vi "Decimation.vi"(10 "d":i32=9, 11 "signal in":waveform(dbl)={"t0"=timestamp(0 s since 1904-01-01), "dt"=9.765625e-08, "Y"=array[2000000 elements]}) -> (3 "output waveform":waveform(dbl)={"t0"=timestamp(0 s since 1904-01-01), "dt"=5e-05, "Y"=array[3907 elements]})   [LabVIEW 2019]
uses:
  MeasSNRResults.ctl
  <vilib>/imath/engines/lvmath2/RunTimeEngine/NodeEndStatement/NIMS_NodeEndStatement_Output.vi
  <instcachedir>/0/NIMS_NodeEndStatement_Output_53EC0D466D134D7ABD903AC30B43404B.lvgen/NIMS_NodeEndStatement_Output_53EC0D466D134D7ABD903AC30B43404B_001.vi
  <vilib>/imath/engines/lvmath2/RunTimeEngine/ErrorHandling/NIMS_Finalize Error.vi
  <vilib>/measure/macond.llb/FIR Filter for 1 Chan.vi
  <vilib>/measure/NI_MAPro.lvlib
panel:
  out "MACS/s Total":dbl
  out "MACS/s 2":dbl=418880000.0
  out "MACS/s":dbl=1423360000.0
  out "MeasSNRResults":T1={"VSignalRMS"=3.2614740031076654e-08, "VNoiseRMS"=0.06936052301211641, "SNR(dB)"=-126.55396876238336, "NumBits"=-21.314612751226473, "SNRFS(dB)"=20.167452857912984, "NumBitsFS"=3.05771642158023} {"SNRFS(dB)" format="%_3p"; "NumBitsFS" format="%.1f"; "NumBits" format="%.1f"; "SNR(dB)" format="%_3p"; "VNoiseRMS" format="%#_3p"; "VSignalRMS" format="%#_3p"}
  out "Fs":dbl=10240000.0
  out "FIR filter specifications 2":T2={"Topology"=enum."FIR by Specification", "Type"=enum."Lowpass", "#Taps"=0, "Lower PB"=9000.0, "Upper PB"=0.0, "Lower SB"=10000.0, "Upper SB"=0.0} {"Lower SB" format="%0.2p"; "Upper SB" format="%0.2p"; "Lower PB" format="%0.2p"; "Upper PB" format="%0.2p"}
  out "filter information 2":T3={"magnitude H(w)"={"f0"=0.0, "df"=312.5, "Mag H(w)"=array[513 elements]}, "phase H(w)"={"f0"=0.0, "df"=312.5, "Phase H(w)"=array[513 elements]}, "order"=1309} {"phase H(w)"."df" format="%.2p"; "phase H(w)"."f0" format="%.2p"; "phase H(w)"."Phase H(w)" format="%.2p"; "magnitude H(w)"."df" format="%.2p"; "magnitude H(w)"."f0" format="%.2p"; "magnitude H(w)"."Mag H(w)" format="%.2p"}
  in  "optional FIR filter specifications 2":T4={"PB Gain"=0.087, "SB Gain"=-112.0, "Scale"=TRUE, "Window"=enum."None"} {"SB Gain" format="%.2p"; "PB Gain" format="%.2p"}
  out "filter information":T3={"magnitude H(w)"={"f0"=0.0, "df"=10000.0, "Mag H(w)"=array[513 elements]}, "phase H(w)"={"f0"=0.0, "df"=10000.0, "Phase H(w)"=array[513 elements]}, "order"=139} {"phase H(w)"."df" format="%.2p"; "phase H(w)"."f0" format="%.2p"; "phase H(w)"."Phase H(w)" format="%.2p"; "magnitude H(w)"."df" format="%.2p"; "magnitude H(w)"."f0" format="%.2p"; "magnitude H(w)"."Mag H(w)" format="%.2p"}
  in  "optional FIR filter specifications":T4={"PB Gain"=0.086, "SB Gain"=-112.0, "Scale"=TRUE, "Window"=enum."None"} {"SB Gain" format="%.2p"; "PB Gain" format="%.2p"}
  out "FIR filter specifications":T2={"Topology"=enum."FIR by Specification", "Type"=enum."Lowpass", "#Taps"=0, "Lower PB"=10000.0, "Upper PB"=0.0, "Lower SB"=310000.0, "Upper SB"=0.0} {"Lower SB" format="%0.2p"; "Upper SB" format="%0.2p"; "Lower PB" format="%0.2p"; "Upper PB" format="%0.2p"}
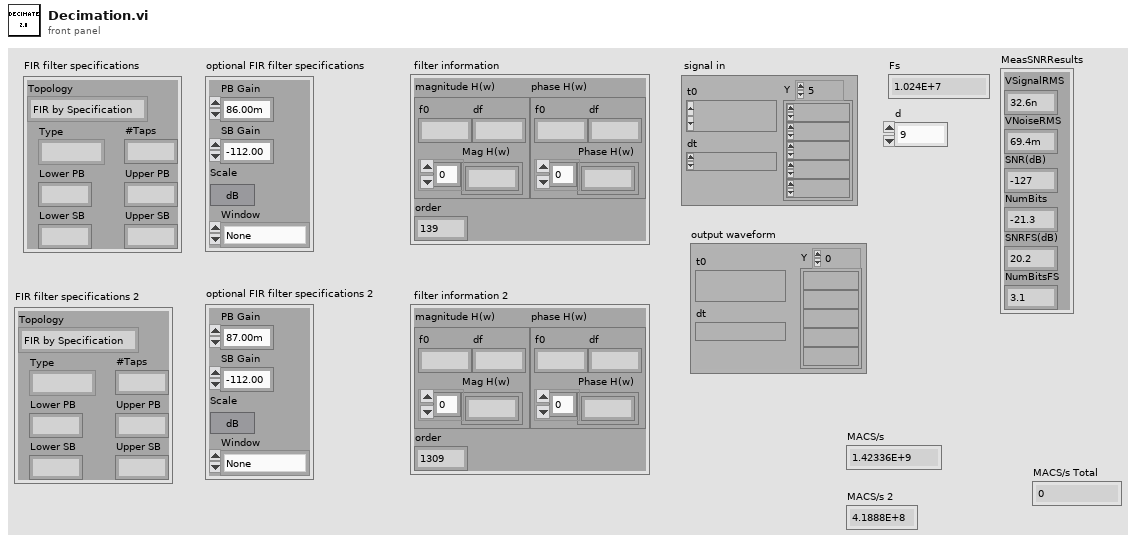
[diagram p1: front panel]
types:
  T1 = typedef "MeasSNRResults.ctl" = cluster{"VSignalRMS":dbl, "VNoiseRMS":dbl, "SNR(dB)":dbl, "NumBits":dbl, "SNRFS(dB)":dbl, "NumBitsFS":dbl}
  T2 = cluster{"Topology":enum16{"Off", "FIR by Specification", "Equi-ripple FIR", "Windowed FIR"}, "Type":enum16{"Lowpass", "Highpass", "Bandpass", "Bandstop"}, "#Taps":i32, "Lower PB":dbl, "Upper PB":dbl, "Lower SB":dbl, "Upper SB":dbl}
  T3 = cluster{"magnitude H(w)":cluster{"f0":dbl, "df":dbl, "Mag H(w)":dbl[]}, "phase H(w)":cluster{"f0":dbl, "df":dbl, "Phase H(w)":dbl[]}, "order":i32}
  T4 = cluster{"PB Gain":dbl, "SB Gain":dbl, "Scale":bool, "Window":enum16{"None", "Hanning", "Hamming", "Triangular", "Blackman", "Exact Blackman", "Blackman-Harris", "Kaiser-Bessel", "Flat Top"}}
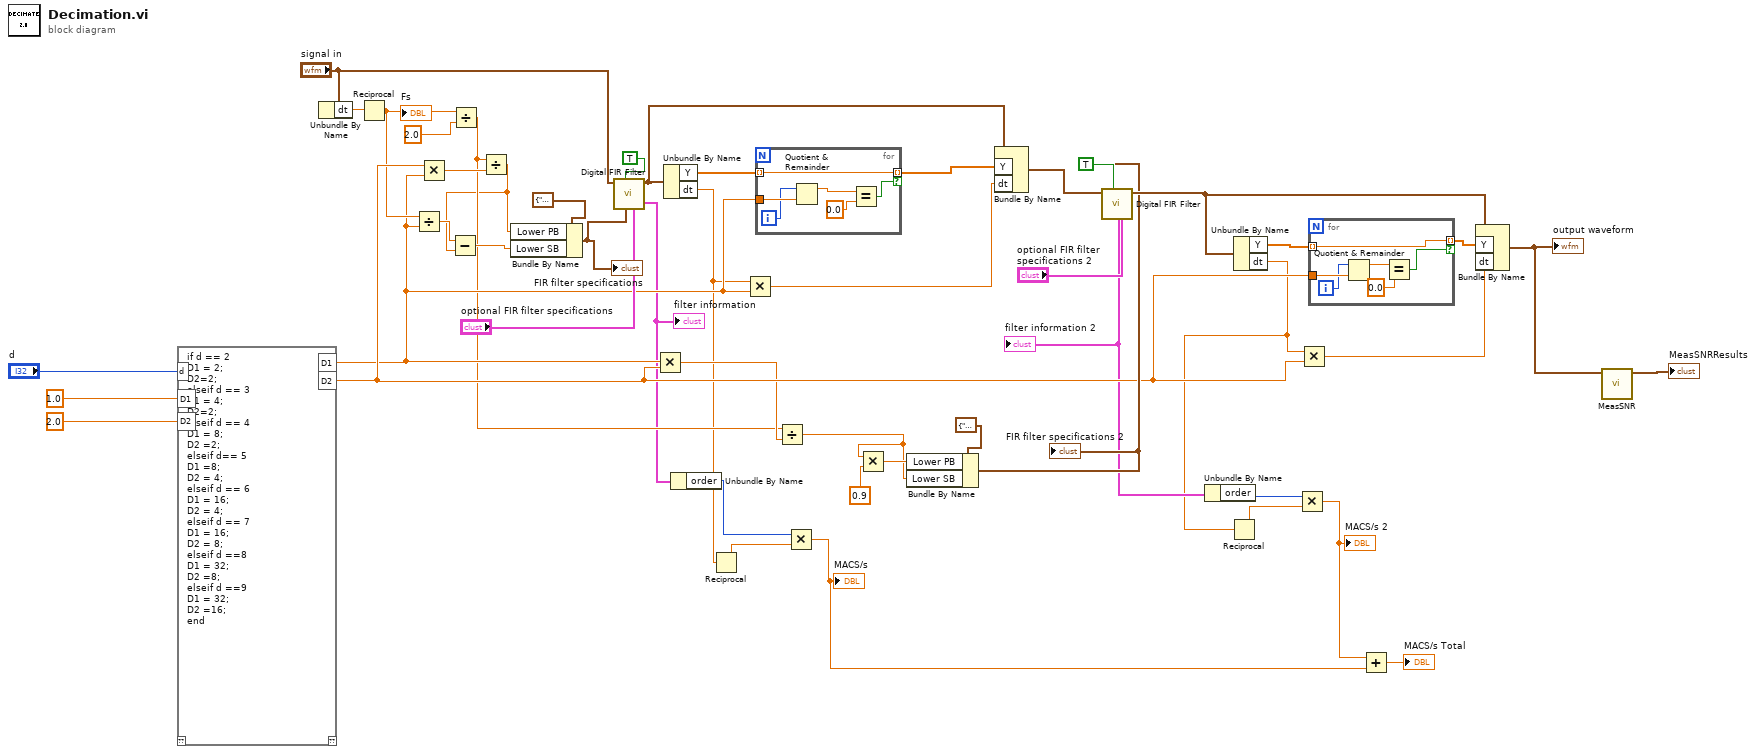
[diagram p0: block diagram]
diagram:
  n1 = mathscript code="if d == 2\nD1 = 2;\nD2=2;\nelseif d == 3\nD1 = 4;\nD2=2;\nelseif d == 4\nD1 = 8;\nD2 =2;\nelseif d== 5\nD1 =8;\nD2 = 4;\nelseif d == 6\nD1 = 16;\nD2 = 4;\nelseif d == 7\nD1 = 16;\nD2 = 8;\nelseif d ==8\nD1 = 32;\nD2 =8;\nelseif d ==9\nD1 = 32;\nD2 =16;\nend"("d"="d", "D1"=1.0, "D2"=2.0) -> ("D1"=w17:dbl, "D2"=w27:dbl)  [unwired: 1 in, 1 out]
  n2 = Unbundle By Name("signal in") -> ("dt"=w21:dbl)
  n3 = Reciprocal(x=w21) -> (1/x=w18:dbl)
  "Fs" <- w18
  n4 = Divide(x=w18, y=w17) -> (x/y=w29:dbl)
  n5 = Multiply(x=w27, y=w17) -> (x*y=w31:dbl)
  n6 = Divide(x=w18, y=2.0) -> (x/y=w16:dbl)
  n7 = Divide(x=w16, y=w31) -> (x/y=w15:dbl)
  n8 = Subtract(x=w29, y=w15) -> (x-y=w28:dbl)
  n9 = Bundle By Name(cluster=T2 {"Topology"=enum."FIR by Specification", "Type"=enum."Lowpass", "#Taps"=0, "Lower PB"=100.0, "Upper PB"=0.0, "Lower SB"=0.0, "Upper SB"=0.0} ("FIR filter specifications"), "Lower PB"=w15, "Lower SB"=w28) -> (w30:T2)
  "FIR filter specifications" <- w30
  n10 = call-poly <vilib>:"Digital FIR Filter.vi"("optional FIR filter specifications"="optional FIR filter specifications", "FIR filter specifications"=w30, "reset filter"=TRUE, "signal in"="signal in") -> ("filter information"=w11:T3, "signal out"=w12:waveform(dbl))  [unwired: 5 in, 1 out]
  "filter information" <- w11
  n11 = Multiply(x=w17, y=w27) -> (x*y=w19:dbl)
  n12 = Unbundle By Name(w12) -> ("Y"=w40:dbl[], "dt"=w10:dbl)
  n13 = Unbundle By Name(w11) -> ("order"=w9:i32)
  n14 = Reciprocal(x=w10) -> (1/x=w8:dbl)
  n15 = Multiply(x=w10, y=w17) -> (x*y=w38:dbl)
  n16 = for {
    tunnel: w40 -> [w50] mode=indexing
    tunnel: [w50] -> w39 mode=indexing if=w52
    tunnel: w17 -> [w51]
    i -> [w49]
    n17 = Quotient & Remainder(x=w49, y=w51) -> (x-y*floor(x/y)=w54:dbl)  [unwired: 1 out]
    n18 = Equal?(x=w54, y=0.0) -> (x = y?=w52:bool)
  }
  n19 = Divide(x=w16, y=w19) -> (x/y=w32:dbl)
  n20 = Multiply(x=w9, y=w8) -> (x*y=w2:dbl)
  "MACS/s" <- w2
  n21 = Multiply(x=w32, y=0.9) -> (x*y=w33:dbl)
  n22 = Bundle By Name(cluster=T2 {"Topology"=enum."FIR by Specification", "Type"=enum."Lowpass", "#Taps"=0, "Lower PB"=100.0, "Upper PB"=0.0, "Lower SB"=0.0, "Upper SB"=0.0} ("FIR filter specifications"), "Lower PB"=w33, "Lower SB"=w32) -> (w35:T2)
  "FIR filter specifications 2" <- w35
  n23 = Bundle By Name(cluster=w12, "Y"=w39, "dt"=w38) -> (w26:waveform(dbl))
  n24 = call-poly <vilib>:"Digital FIR Filter.vi"("optional FIR filter specifications"="optional FIR filter specifications 2", "FIR filter specifications"=w35, "reset filter"=TRUE, "signal in"=w26) -> ("filter information"=w5:T3, "signal out"=w43:waveform(dbl))  [unwired: 5 in, 1 out]
  "filter information 2" <- w5
  n25 = Unbundle By Name(w5) -> ("order"=w6:i32)
  n26 = Unbundle By Name(w43) -> ("Y"=w37:dbl[], "dt"=w4:dbl)
  n27 = Reciprocal(x=w4) -> (1/x=w7:dbl)
  n28 = Multiply(x=w6, y=w7) -> (x*y=w3:dbl)
  "MACS/s 2" <- w3
  n29 = Multiply(x=w4, y=w27) -> (x*y=w44:dbl)
  n30 = for {
    tunnel: [w56] -> w36 mode=indexing if=w58
    tunnel: w37 -> [w56] mode=indexing
    tunnel: w27 -> [w57]
    i -> [w55]
    n31 = Quotient & Remainder(x=w55, y=w57) -> (x-y*floor(x/y)=w60:dbl)  [unwired: 1 out]
    n32 = Equal?(x=w60, y=0.0) -> (x = y?=w58:bool)
  }
  n33 = Add(x=w3, y=w2) -> (x+y=→"MACS/s Total":dbl)
  n34 = Bundle By Name(cluster=w43, "Y"=w36, "dt"=w44) -> (w14:waveform(dbl))
  "output waveform" <- w14
  n35 = call "MeasSNR.vi"("Input"=w14) -> ("MeasSNRResults"=→"MeasSNRResults":T1)  [unwired: 9 in, 1 out]
